vi "AddTest.vi"(8 "error in (no error)":errorcluster) -> (0 "error out":errorcluster)   [LabVIEW 2021]
uses:
  <vilib>/addons/_JKI Toolkits/Caraya/classes/Test/Test.lvclass
  <vilib>/addons/_JKI Toolkits/Caraya/classes/Assert/Assert.lvclass
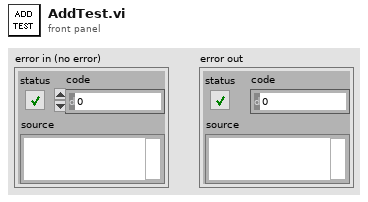
[diagram p1: front panel]
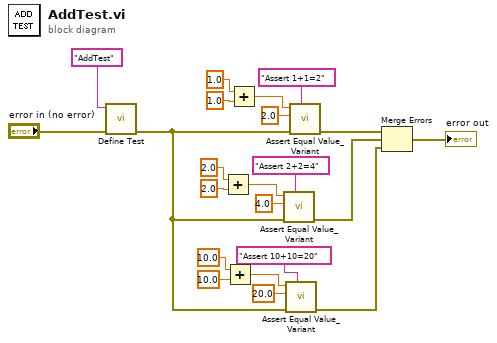
[diagram p0: block diagram]
diagram:
  n1 = call <vilib>:"Define Test.vi"("error in (no error)"="error in (no error)", "Label (VI Title)"="AddTest") -> ("error out"=w2:errorcluster)  [unwired: 8 in, 1 out]
  n2 = Add(x=2.0, y=2.0) -> (x+y=w12:dbl)
  n3 = Add(x=10.0, y=10.0) -> (x+y=w6:dbl)
  n4 = Add(x=1.0, y=1.0) -> (x+y=w21:dbl)
  n5 = call <vilib>:"Assert Equal Value_Variant.vi"("Label"="Assert 2+2=4", "error in (no error)"=w2, "Y"=4.0 ("y"), "X"=w12) -> ("error out"=w8:errorcluster)  [unwired: 6 in, 1 out]
  n6 = call <vilib>:"Assert Equal Value_Variant.vi"("Label"="Assert 10+10=20", "error in (no error)"=w2, "Y"=20.0 ("y"), "X"=w6) -> ("error out"=w1:errorcluster)  [unwired: 6 in, 1 out]
  n7 = call <vilib>:"Assert Equal Value_Variant.vi"("Label"="Assert 1+1=2", "error in (no error)"=w2, "Y"=2.0 ("y"), "X"=w21) -> ("error out"=w10:errorcluster)  [unwired: 6 in, 1 out]
  n8 = Merge Errors(w10, w8, w1) -> (→"error out":errorcluster)
